vi "readsignal_lowpass.vi"() -> ()   [LabVIEW 2023]
uses:
  <vilib>/addons/Biomedical/Biosignal Measurements/EEG/EEG FFT Spectrum (Waveform).vi
  <vilib>/addons/Biomedical/NI_BMTK_Measurements.lvlib
panel:
  out "Output Waveform":waveform(dbl)
  out "EEG Signal":waveform(dbl)(graph)
  in  "dt":dbl format="%#_7f"
  in  "t0":timestamp
  in  "Waveform":waveform(dbl)
  in  "format string":string
  in  "array type (2D Dbl)":dbl[][](array[numeric])
  in  "file (use dialog)":path
  out "Gamma Wave FFT Spectrum":cluster{"f0":dbl, "df":dbl, "S(f)":dbl[]}(graph)
  out "Beta Wave FFT Spectrum":cluster{"f0":dbl, "df":dbl, "S(f)":dbl[]}(graph)
  out "Alpha Wave FFT Spectrum":cluster{"f0":dbl, "df":dbl, "S(f)":dbl[]}(graph)
  out "Theta Wave FFT Spectrum":cluster{"f0":dbl, "df":dbl, "S(f)":dbl[]}(graph)
  out "Delta Wave FFT Spectrum":cluster{"f0":dbl, "df":dbl, "S(f)":dbl[]}(graph)
  out "FFT Spectrum":cluster{"f0":dbl, "df":dbl, "S(f)":dbl[]}(graph)
  out "Delta Wave":dynamicdata(graph)
  out "Gamma Wave":dynamicdata(graph)
  out "Beta Wave":dynamicdata(graph)
  out "Alpha Wave":dynamicdata(graph)
  out "Theta Wave":dynamicdata(graph)
  out "Saída do High-pass 1Hz":dynamicdata(graph)
  out "Saída do Low-pass 31Hz":dynamicdata(graph)
  out "After Low-pass: fc = 40 Hz":dynamicdata(graph)
  in  "stop":bool
  # "0,0019531"
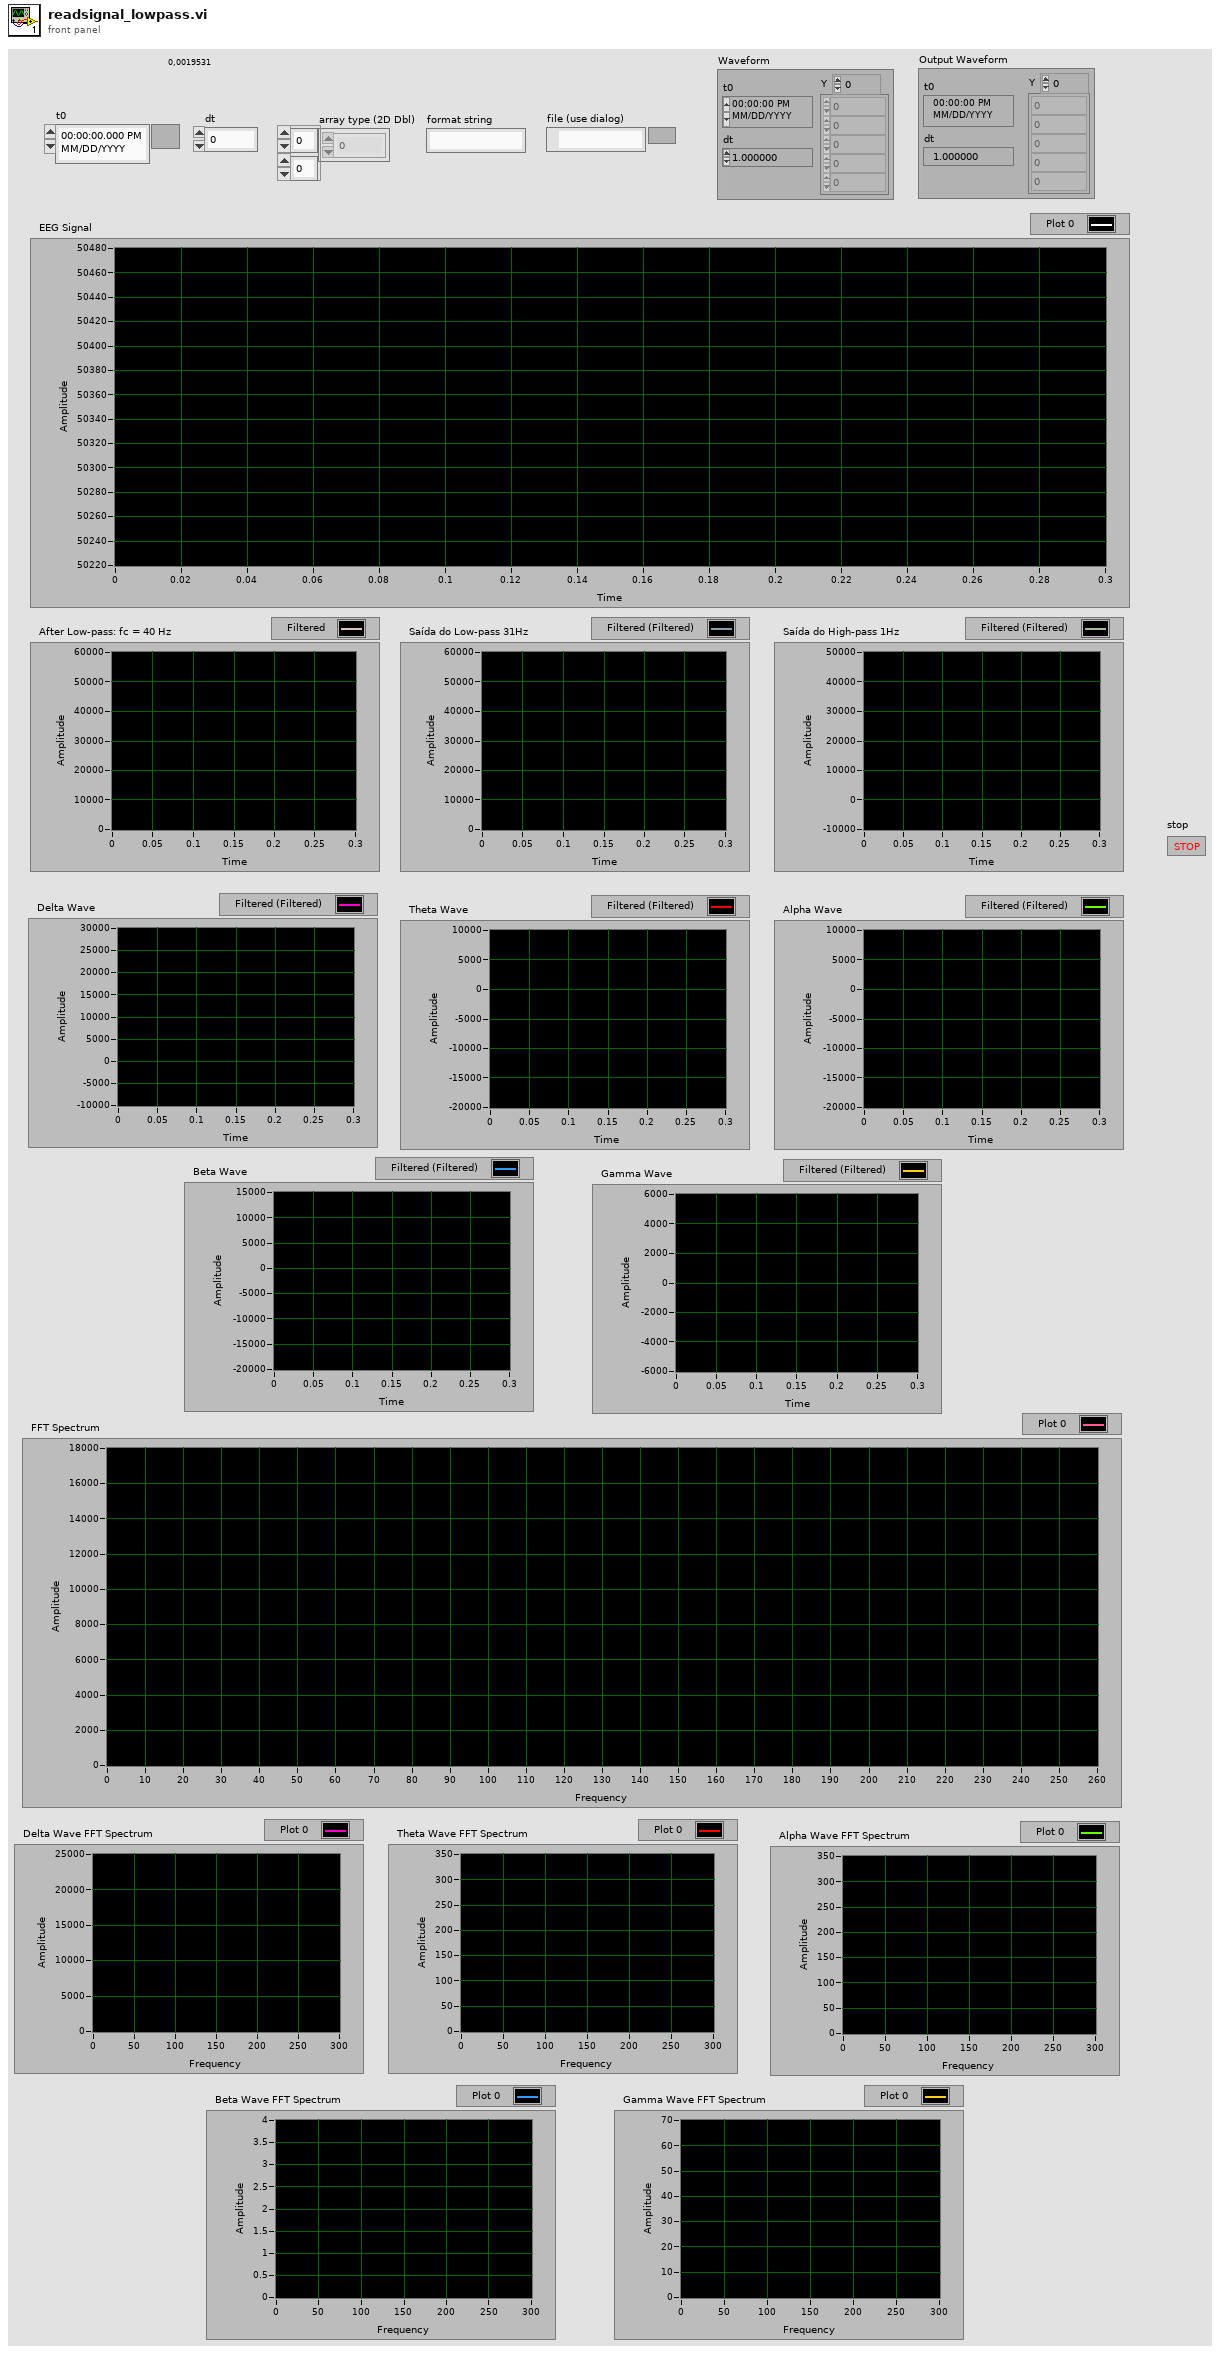
[diagram p1: front panel]
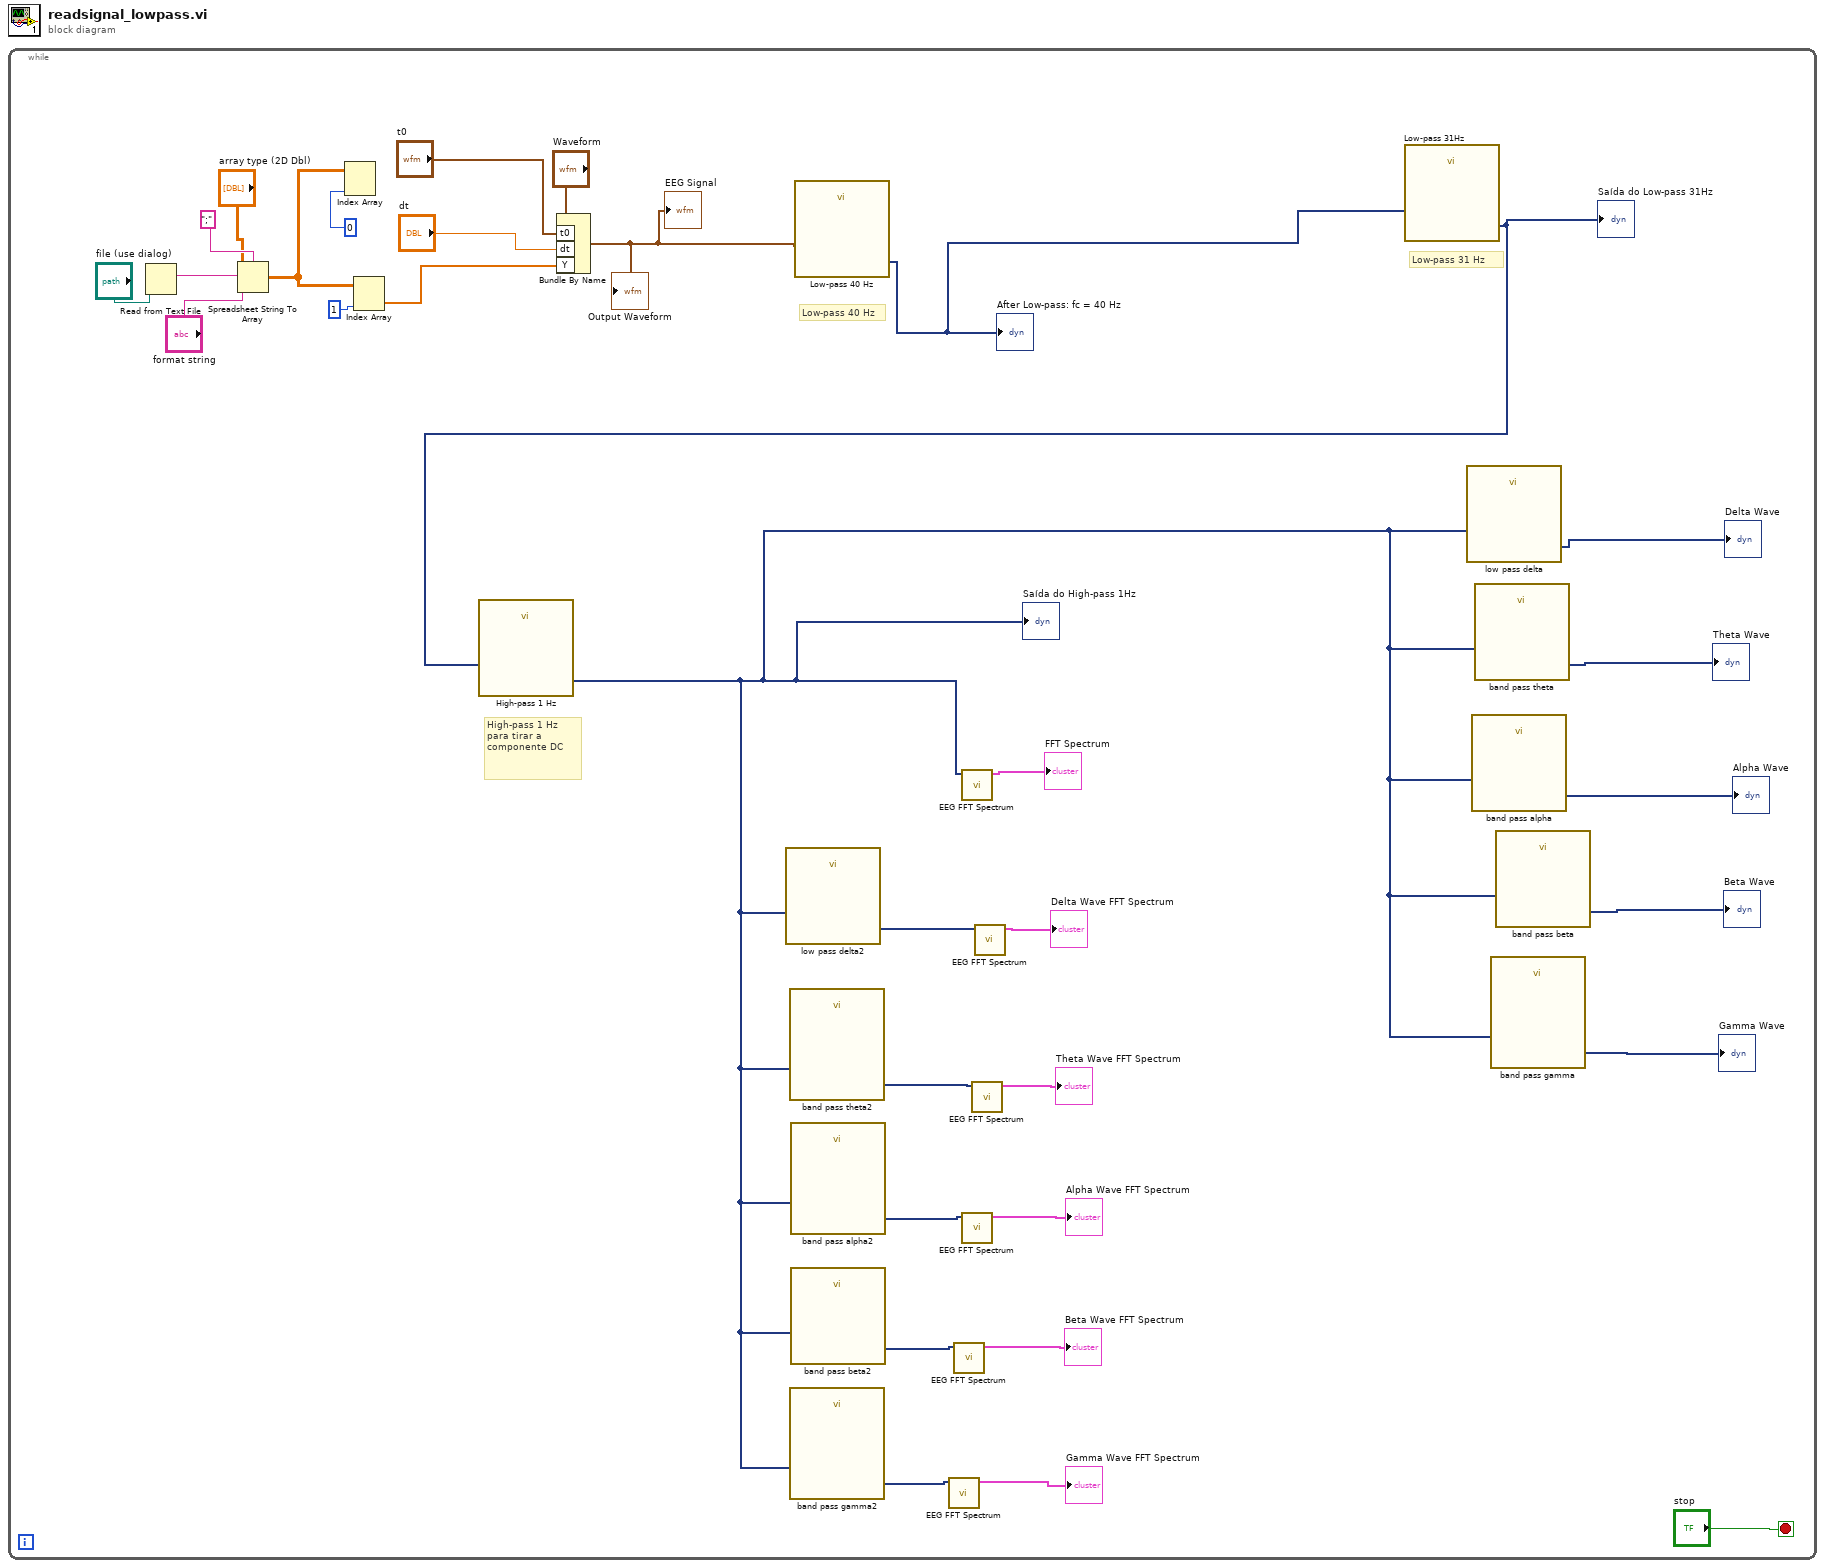
[diagram p0: block diagram]
diagram:
  n1 = while {
    stop <- "stop" stop-if-true
    # "Low-pass 40 Hz"
    # "High-pass 1 Hz para tirar a componente DC"
    # "Low-pass 31 Hz"
    n2 = Read from Text File(file (use dialog)="file (use dialog)") -> (text=w9:string)  [unwired: 3 in, 3 out]
    n3 = Spreadsheet String To Array(delimiter (Tab)=";", format string="format string", spreadsheet string=w9, array type (2D Dbl)="array type (2D Dbl)") -> (array=w13:dbl[][])
    n4 = Index Array(array=w13, index (col)=0 ("disabled index (col)")) -> ()  [unwired: 1 in, 1 out]
    n5 = Index Array(array=w13, index (col)=1 ("disabled index (col)")) -> (element=w6:dbl[])  [unwired: 1 in]
    n6 = Bundle By Name(cluster="Waveform", "t0"="t0", "dt"="dt", "Y"=w6) -> (w2:waveform(dbl))
    "EEG Signal" <- w2
    "Output Waveform" <- w2
    n7 = call "Low-pass 40 Hz"("Signal"=w2) -> ("Filtered Signal"=w1:dynamicdata)  [unwired: 9 in, 1 out]
    "After Low-pass: fc = 40 Hz" <- w1
    n8 = call "Low-pass 31Hz"("Signal"=w1) -> ("Filtered Signal"=w32:dynamicdata)  [unwired: 9 in, 1 out]
    "Saída do Low-pass 31Hz" <- w32
    n9 = call "High-pass 1 Hz"("Signal"=w32) -> ("Filtered Signal"=w25:dynamicdata)  [unwired: 9 in, 1 out]
    "Saída do High-pass 1Hz" <- w25
    n10 = call "low pass delta2"("Signal"=w25) -> ("Filtered Signal"=w23:dynamicdata)  [unwired: 9 in, 1 out]
    n11 = call "band pass theta2"("Signal"=w25) -> ("Filtered Signal"=w22:dynamicdata)  [unwired: 9 in, 1 out]
    n12 = call "band pass gamma2"("Signal"=w25) -> ("Filtered Signal"=w15:dynamicdata)  [unwired: 9 in, 1 out]
    n13 = call "band pass alpha2"("Signal"=w25) -> ("Filtered Signal"=w19:dynamicdata)  [unwired: 9 in, 1 out]
    n14 = call "band pass beta2"("Signal"=w25) -> ("Filtered Signal"=w17:dynamicdata)  [unwired: 9 in, 1 out]
    n15 = call-poly <vilib>:"EEG FFT Spectrum.vi"("EEG"=w15) -> ("FFT spectrum"=→"Gamma Wave FFT Spectrum":cluster{"f0":dbl, "df":dbl, "S(f)":dbl[]})  [unwired: 8 in, 2 out]
    n16 = call-poly <vilib>:"EEG FFT Spectrum.vi"("EEG"=w17) -> ("FFT spectrum"=→"Beta Wave FFT Spectrum":cluster{"f0":dbl, "df":dbl, "S(f)":dbl[]})  [unwired: 8 in, 2 out]
    n17 = call-poly <vilib>:"EEG FFT Spectrum.vi"("EEG"=w25) -> ("FFT spectrum"=→"FFT Spectrum":cluster{"f0":dbl, "df":dbl, "S(f)":dbl[]})  [unwired: 8 in, 2 out]
    n18 = call-poly <vilib>:"EEG FFT Spectrum.vi"("EEG"=w19) -> ("FFT spectrum"=→"Alpha Wave FFT Spectrum":cluster{"f0":dbl, "df":dbl, "S(f)":dbl[]})  [unwired: 8 in, 2 out]
    n19 = call-poly <vilib>:"EEG FFT Spectrum.vi"("EEG"=w22) -> ("FFT spectrum"=→"Theta Wave FFT Spectrum":cluster{"f0":dbl, "df":dbl, "S(f)":dbl[]})  [unwired: 8 in, 2 out]
    n20 = call-poly <vilib>:"EEG FFT Spectrum.vi"("EEG"=w23) -> ("FFT spectrum"=→"Delta Wave FFT Spectrum":cluster{"f0":dbl, "df":dbl, "S(f)":dbl[]})  [unwired: 8 in, 2 out]
    n21 = call "low pass delta"("Signal"=w25) -> ("Filtered Signal"=→"Delta Wave":dynamicdata)  [unwired: 9 in, 1 out]
    n22 = call "band pass alpha"("Signal"=w25) -> ("Filtered Signal"=→"Alpha Wave":dynamicdata)  [unwired: 9 in, 1 out]
    n23 = call "band pass theta"("Signal"=w25) -> ("Filtered Signal"=→"Theta Wave":dynamicdata)  [unwired: 9 in, 1 out]
    n24 = call "band pass gamma"("Signal"=w25) -> ("Filtered Signal"=→"Gamma Wave":dynamicdata)  [unwired: 9 in, 1 out]
    n25 = call "band pass beta"("Signal"=w25) -> ("Filtered Signal"=→"Beta Wave":dynamicdata)  [unwired: 9 in, 1 out]
  }
